vi "fpga_write_parameters.vi"(6 "Ramp parameters XY":T1, 7 "FPGA_acquisition_parameters":T6, 8 "error in":errorcluster, 9 "FPGA Scan Parameters":T8={"No. of waveforms"=11, "Continuous scanning"=TRUE}, 10 "FPGA Cycle Parameters XY":T9={"Cycle parameters X"={"Imaging cycles"=285714, "Settling cycles"=71429, "Resting cycles"=42857, "Phase advance per cycle"=0.0001399517059326172, "Initial Phase"=0.00286865234375}, "Cycle parameters Y"={"Imaging cycles"=285714, "Settling cycles"=71429, "Resting cycles"=42857, "Phase advance per cycle"=0.0001399517059326172, "Initial Phase"=0.00286865234375}}, 11 "FPGA VI Reference in":T7) -> (0 "error out":errorcluster, 3 "FPGA VI Reference Out":T7)   [LabVIEW 2011, in "Fiberscope_library.lvlib"]
uses:
  Fiberscope_library.lvlib
  typedefs/fpga_main_spiral_fpga_ref.ctl
  fpga/typedefs/cycle_parameters_XY_cluster.ctl
  fpga/typedefs/cycle_parameters_cluster.ctl
  fpga/typedefs/scan_parameters_cluster.ctl
  typedefs/FPGA_acquisition_parameters.ctl
  fpga/typedefs/ramp_parameters_XY_cluster.ctl
  fpga/typedefs/ramp_parameters_cluster.ctl
  fpga/typedefs/ramp_type_enum.ctl
  fpga/typedefs/linear_ramp_parameters_cluster.ctl
  fpga/typedefs/sine_ramp_parameters_cluster.ctl
  <vilib>/Utility/error.llb/Error Cluster From Error Code.vi
  <vilib>/rvi/errors/niLvFpgaAdjustHostInterfaceError.vi
  <vilib>/rvi/interface/nirviReadWriteControl/nirviReadWriteControl.xnode
  FPGA Bitfiles/FiberscopeRK1107_FPGATarget_fpgamainspiral_0DF2A7CB.lvbitx
  NiFpgaLv.dll
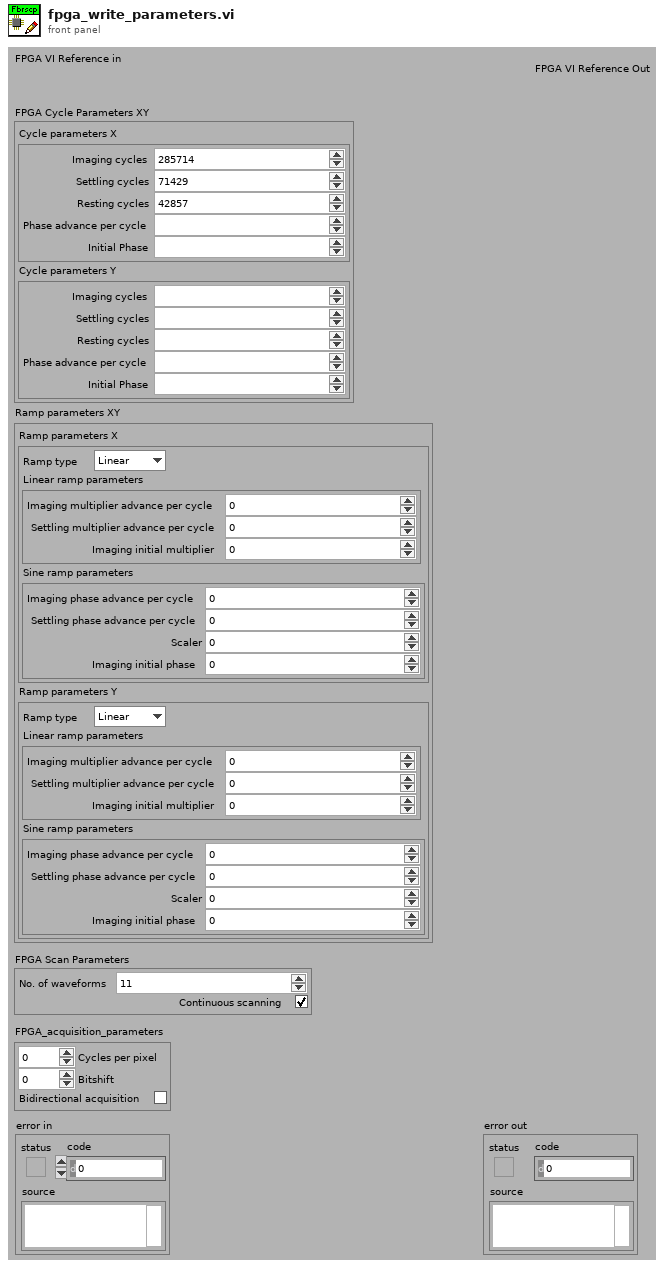
[diagram p1: front panel]
types:
  T1 = typedef "ramp_parameters_XY_cluster.ctl" = cluster{"Ramp parameters X":T2, "Ramp parameters Y":T2}
  T2 = typedef "ramp_parameters_cluster.ctl" = cluster{"Ramp type":T3, "Linear ramp parameters":T4, "Sine ramp parameters":T5}
  T3 = typedef "ramp_type_enum.ctl" = enum8{"Linear", "Sine"}
  T4 = typedef "linear_ramp_parameters_cluster.ctl" = cluster{"Imaging multiplier advance per cycle":fxp<+/-,32,0>, "Settling multiplier advance per cycle":fxp<+/-,32,0>, "Imaging initial multiplier":fxp<+/-,43,12>}
  T5 = typedef "sine_ramp_parameters_cluster.ctl" = cluster{"Imaging phase advance per cycle":fxp<+,32,0>, "Settling phase advance per cycle":fxp<+,32,0>, "Scaler":fxp<+,43,12>, "Imaging initial phase":fxp<+,32,1>}
  T6 = typedef "Fiberscope_library.lvlib/FPGA_acquisition_parameters.ctl" = cluster{"Cycles per pixel":u32, "Bitshift":i8, "Bidirectional acquisition":bool}
  T7 = typedef "Fiberscope_library.lvlib/fpga_main_spiral_fpga_ref.ctl" = refnum<k20>
  T8 = typedef "scan_parameters_cluster.ctl" = cluster{"No. of waveforms":u16, "Continuous scanning":bool}
  T9 = typedef "cycle_parameters_XY_cluster.ctl" = cluster{"Cycle parameters X":T10, "Cycle parameters Y":T10}
  T10 = typedef "cycle_parameters_cluster.ctl" = cluster{"Imaging cycles":i32, "Settling cycles":i32, "Resting cycles":i32, "Phase advance per cycle":fxp<+,32,0>, "Initial Phase":fxp<+,32,1>}
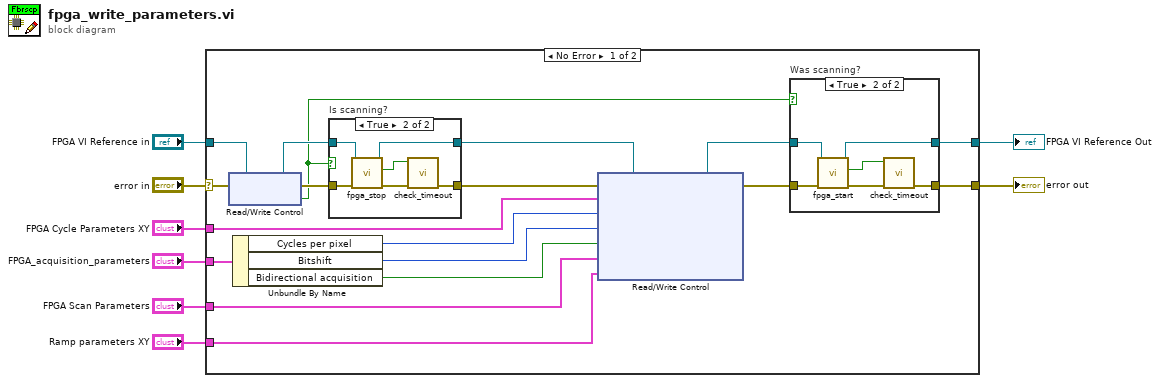
[diagram p0: block diagram]
diagram:
  n1 = case shown="No Error" "error in" {
    selector: "error in" -> [w26 w44]
    tunnel: [w19 w44] -> w7
    tunnel: "FPGA VI Reference in" -> [w25 w43]
    tunnel: "FPGA Cycle Parameters XY" -> [w24 _]
    tunnel: "FPGA_acquisition_parameters" -> [w16 _]
    tunnel: "FPGA Scan Parameters" -> [w11 _]
    tunnel: [w18 w43] -> w3
    tunnel: "Ramp parameters XY" -> [w9 _]
    frame No Error {
      n2 = xnode "Read/Write Control"("FPGA VI Reference In"=w25, "error in"=w26) -> ("FPGA VI Reference Out"=w22:T7, "error out"=w23:errorcluster, "Scanning?"=w17:bool)
      n3 = Unbundle By Name(w16) -> ("Cycles per pixel"=w13:u32, "Bitshift"=w12:i8, "Bidirectional acquisition"=w10:bool)
      n4 = case "Is scanning?" shown="True" w17 {
        tunnel: w23 -> [w35 w42]
        tunnel: w22 -> [w36 w41]
        tunnel: [w35 w38] -> w21
        tunnel: [w36 w40] -> w20
        frame False {
        }
        frame True {
          n5 = call "fpga_stop.vi"("error in"=w42, "FPGA VI Reference in"=w41) -> ("error out"=w39:errorcluster, "Timed out?"=w37:bool, "FPGA VI Reference out"=w40:T7)  [unwired: 7 in]
          n6 = call "check_timeout.vi"("error in"=w39, "Timeout?"=w37) -> ("error out"=w38:errorcluster)  [unwired: 9 in]
        }
      }
      n7 = xnode "Read/Write Control"("FPGA VI Reference In"=w20, "error in"=w21, "Cycle parameters XY"=w24, "cycles per pixel"=w13, "bitshift"=w12, "Bidirectional acquisition"=w10, "Scan parameters"=w11, "Ramp parameters XY"=w9) -> ("FPGA VI Reference Out"=w15:T7, "error out"=w14:errorcluster)
      n8 = case "Was scanning?" shown="True" w17 {
        tunnel: w14 -> [w27 w34]
        tunnel: [w27 w30] -> w19
        tunnel: w15 -> [w28 w33]
        tunnel: [w28 w32] -> w18
        frame False {
        }
        frame True {
          n9 = call "fpga_start.vi"("error in"=w34, "FPGA VI Reference in"=w33) -> ("error out"=w31:errorcluster, "Timed out?"=w29:bool, "FPGA VI Reference out"=w32:T7)  [unwired: 7 in]
          n10 = call "check_timeout.vi"("error in"=w31, "Timeout?"=w29) -> ("error out"=w30:errorcluster)  [unwired: 9 in]
        }
      }
    }
    frame Error {
    }
  }
  "error out" <- w7
  "FPGA VI Reference Out" <- w3
